vi "RTG_Host_Main.vi"() -> ()   [LabVIEW 2020]
uses:
  <vilib>/RTG/API/interface/public/State.ctl
  <vilib>/RTG/API/ip/common/host-types/Target Configuration.ctl
  <vilib>/RTG/API/ip/common/host-types/Synchronization - Host.ctl
  <vilib>/RTG/API/ip/common/host-types/Synchronization Mode - Host.ctl
  <vilib>/RTG/API/ip/common/host-types/Basic Target - Host.ctl
  <vilib>/RTG/API/ip/common/host-types/Target Motion Parameters.ctl
  <vilib>/RTG/API/ip/common/host-types/Single Target Motion Parameters.ctl
  <vilib>/RTG/API/interface/public/Coprocessor Link Status.ctl
  <vilib>/RTG/coprocessor/host/RTG Coprocessor Link Interface/Public/Coprocessor Status.ctl
  Controls/Enum/Program_Status_Enum.ctl
  Controls/Enum/RTG_Enum.ctl
  Controls/Enum/CoProcessor_Enum.ctl
  Controls/Enum/Supervisor_Enum.ctl
  Controls/Clust/RTG Clust.ctl
  <vilib>/RTG/API/interface/NI-RTG Interface.lvclass
  <vilib>/RTG/coprocessor/host/RTG Coprocessor Link Interface/RTG Coprocessor Link Interface.lvclass
  Controls/Clust/RTG API Clust.ctl
  support/Options - API Mode.ctl
  support/Options - Calibration.ctl
  support/Options - Remote.ctl
  <vilib>/Utility/error.llb/Error Cluster From Error Code.vi
  <vilib>/rvi/errors/niLvFpgaAdjustHostInterfaceError.vi
  <vilib>/rvi/interface/nirviReadWriteControl/nirviReadWriteControl.xnode
  RTG Examples.lvlib
  <vilib>/RTG/API/ip/common/host-types/Host Data Types v1.lvlib
  NiFpgaLv.dll
  <vilib>/rvi/interface/Simulation/niFpgaSimulationCallBeginRW.vi
panel:
  out "CoPr":i32
  out "RTG":i32
  out "Spvsr":i32
  out "Spvsr":T1=enum."Spvsr_InitCtrls"
  out "CoPr":T2
  out "RTG":T3
  out "App Status":T4
  in  "Tab Control":T5(tab)
  in  "Instrument Names":string[](array[string])=["5831_0"]
  in  "Coprocessor Names":string[](array[string])
  in  "Center Freqeuncies (Hz)":dbl[](array[numeric])=[5500000000.0] format="%#_6p"
  in  "Reference Levels (dBm)":dbl[](array[numeric])=[0.0]
  in  "Calibrate":bool=TRUE
  in  "abort system self cal":bool
  in  "Commit HW":bool
  in  "ExtAtten":dbl[](array[numeric]) caption="External Attenuations (dB)"
  in  "OffsFreq":dbl[](array[numeric]) caption="Offset Frequencies (Hz)" format="%#_6p"
  in  "ExtDelay":dbl[](array[numeric]) caption="External Delay (s)" format="%#_6p"
  in  "mmWave Radio Heads Enable":bool[](array[boolean])
  in  "PRI (s)":dbl[](array[numeric]) format="%#_6p"
  in  "Set PRIs":bool
  out "Min Latencies (s)":dbl[](array[numeric]) format="%#_6p"
  out "Min Common Attenuations (dB)":dbl[](array[numeric])
  out "Max Common Attenuations (dB)":dbl[](array[numeric])
  out "Versions":string[](array[string])
  in  "Common Attenuation (dB)":dbl
  in  "Auto Send Software Trigger":bool
  in  "Prepend Software Trigger":bool
  in  "Device Index":i32
  in  "Target Configuration Files":path[](array[path])
  in  "Target Configuration":T6 {"rtg targets"."time offset (s)" format="%#_6p"; "rtg targets"."doppler" format="%#_6p"}
  in  "Target Motion Parameters":T10={"target motions"=[{"target enable"=FALSE, "start time offset (s)"=-1e-09, "time offset rate of change (s/s)"=0.001, "start attenuation (dB)"=0.0, "attenuation rate of change (dB/s)"=0.0, "start frequency shift (Hz)"=0.0, "frequency shift rate of change (Hz/sec)"=0.0}], "scenario duration (s)"=67.0, "configuration update rate(Hz)"=15000.0} {"configuration update rate(Hz)" format="%#_6p"; "target motions"."frequency shift rate of change (Hz/sec)" format="%#_6p"; "target motions"."start frequency shift (Hz)" format="%#_6p"; "target motions"."time offset rate of change (s/s)" format="%#_6p"; "target motions"."start time offset (s)" format="%#_6p"}
  in  "Send TrgtCfg":bool
  in  "Send Motion":bool
  in  "Send Files":bool
  in  "Start RTG":bool
  in  "Stop RTG":bool
  in  "Send SW Trigg":bool
  out "rtg link status":T12[](array[typedef])
  out "Trigger Count":i32[][](array[numeric]) caption="Device Index vs Trigger Count"
  out "RTG Status":string
  out "RTG State":T13
  out "error out":errorcluster
  out "System Time":string
  out "coproc link":T14[](array[typedef]) caption="coprocessor link status"
  in  "Exit":bool
  # "v20230901"
  # "Configuration Files and Target Motion"
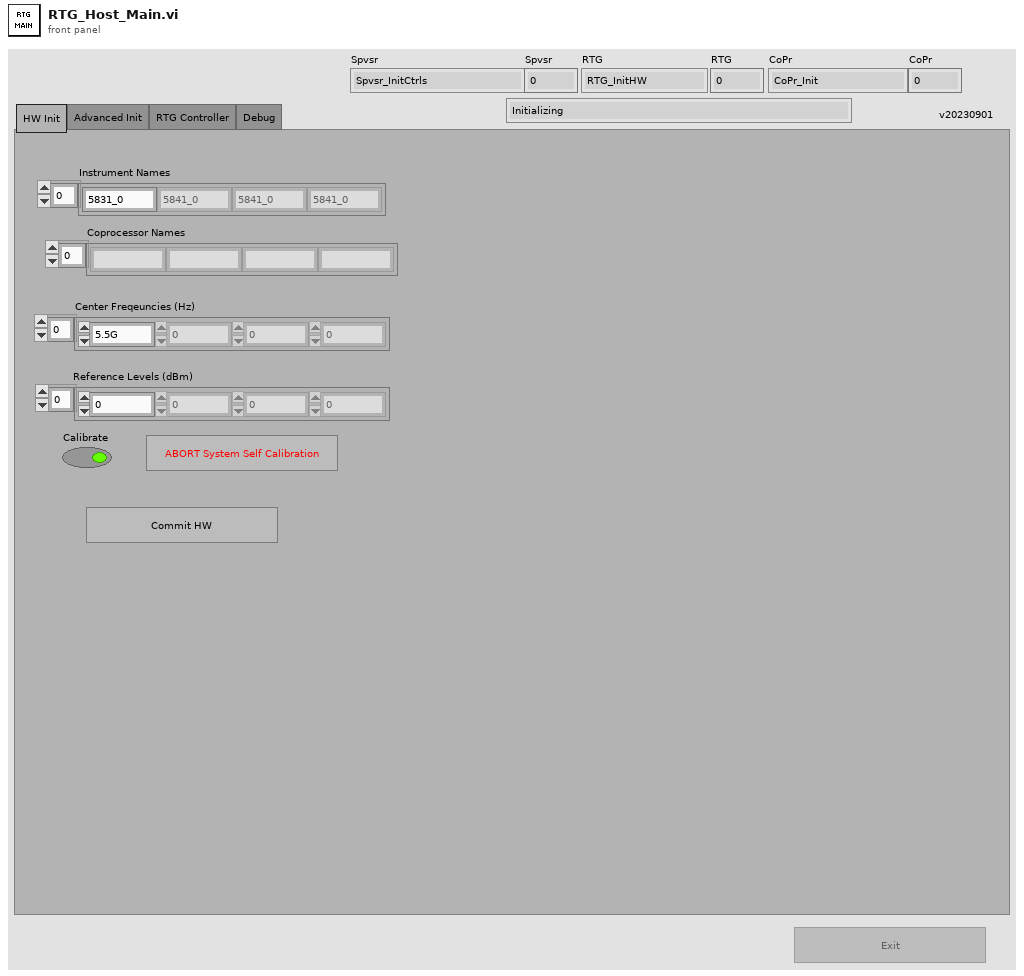
[diagram p1: front panel]
types:
  T1 = typedef "Supervisor_Enum.ctl" = enum16{"Spvsr_InitSW", "Spvsr_InitCtrls", "Spvsr_UpdtFP", "Spvsr_InitRTG", "Spvsr_StateCount", "Spvsr_Exit"}
  T2 = typedef "CoProcessor_Enum.ctl" = enum16{"CoPr_Init", "CoPr_Chk", "CoPr_Exit"}
  T3 = typedef "RTG_Enum.ctl" = enum16{"RTG_InitHW", "RTG_RefLvl", "RTG_mmWav", "RTG_Cal", "RTG_CalDone?", "RTG_ExtAtten", "RTG_GetCal", "RTG_SetPRIs", "RTG_CommAtten", "RTG_TargetSetup", "RTG_Send Files", "RTG_Send Target Cfg", "RTG_Send Motion", "RTG_Send SW Trigg", "RTG_Start", "RTG_Stop", "RTG_Chk", "RTG_Exit"}
  T4 = typedef "Program_Status_Enum.ctl" = enum16{"Initializing", "RTG Inactive", "Unconfigured", "RTG active", "Error", "Closing", "Closed"}
  T5 = enum32{"HW Init", "Advanced Init", "RTG Controller", "Debug"}
  T6 = typedef "Host Data Types v1.lvlib/Target Configuration.ctl" = cluster{"synchronization":T7, "rtg targets":T9[]}
  T7 = typedef "Host Data Types v1.lvlib/Synchronization - Host.ctl" = cluster{"synch mode":T8, "time offset (s)":dbl}
  T8 = typedef "Host Data Types v1.lvlib/Synchronization Mode - Host.ctl" = enum16{"Software Trigger", "Hardware Trigger", "Time Offset Relative to First", "Time Offset Relative to Last", "Pulse Rising Edge", "Pulse Falling Edge"}
  T9 = typedef "Host Data Types v1.lvlib/Basic Target - Host.ctl" = cluster{"time offset (s)":dbl, "attenuaton (dB)":dbl, "doppler":dbl, "target enable":bool, "relative velocity enable":bool}
  T10 = typedef "Host Data Types v1.lvlib/Target Motion Parameters.ctl" = cluster{"target motions":T11[], "scenario duration (s)":dbl, "configuration update rate(Hz)":dbl}
  T11 = typedef "Host Data Types v1.lvlib/Single Target Motion Parameters.ctl" = cluster{"target enable":bool, "start time offset (s)":dbl, "time offset rate of change (s/s)":dbl, "start attenuation (dB)":dbl, "attenuation rate of change (dB/s)":dbl, "start frequency shift (Hz)":dbl, "frequency shift rate of change (Hz/sec)":dbl}
  T12 = typedef "NI-RTG v1.lvlib/NI-RTG Interface.lvclass/Coprocessor Link Status.ctl" = cluster{"task name":string, "device name":string, "hard error":bool, "soft error":bool, "channel up":bool, "system reset":bool}
  T13 = typedef "NI-RTG v1.lvlib/NI-RTG Interface.lvclass/State.ctl" = enum16{"Idle", "Inactive", "Active", "System Self Calibration"}
  T14 = typedef "RTG Coprocessor Link Interface v1 Host.lvlib/RTG Coprocessor Link Interface.lvclass/Coprocessor Status.ctl" = cluster{"tx read count":u64, "tx read overflow":bool, "rx read count":u64, "rx read overflow":bool}
  T15 = cluster{"CoPr Refs":refnum<class "RTG Coprocessor Link Interface.lvclass">[]}
  T16 = typedef "RTG Clust.ctl" = cluster{"VST_Names":string[], "OptionString":string, "RTG Ref":refnum<class "NI-RTG Interface.lvclass">, "Index":i32, "AutoSend":bool, "Prepend":bool, "state":T13}
  T17 = enum8{"Enabled", "Disabled", "Disabled and Grayed Out"}
  T18 = typedef "RTG API Clust.ctl" = cluster{"Local?":T19, "Cal":T20, "Remote":T21, "ini path":path}
  T19 = typedef "RTG Examples.lvlib/Options - API Mode.ctl" = enum16{"Local", "Remote"}
  T20 = typedef "RTG Examples.lvlib/Options - Calibration.ctl" = cluster{"enable internal loopback  ":bool, "enable overwrite cal data  ":bool, "enable save cal data           ":bool, "disable self cal range          ":bool}
  T21 = typedef "RTG Examples.lvlib/Options - Remote.ctl" = cluster{"ip address":string, "port":string, "certificate path":path, "timeout (ms)":i32}
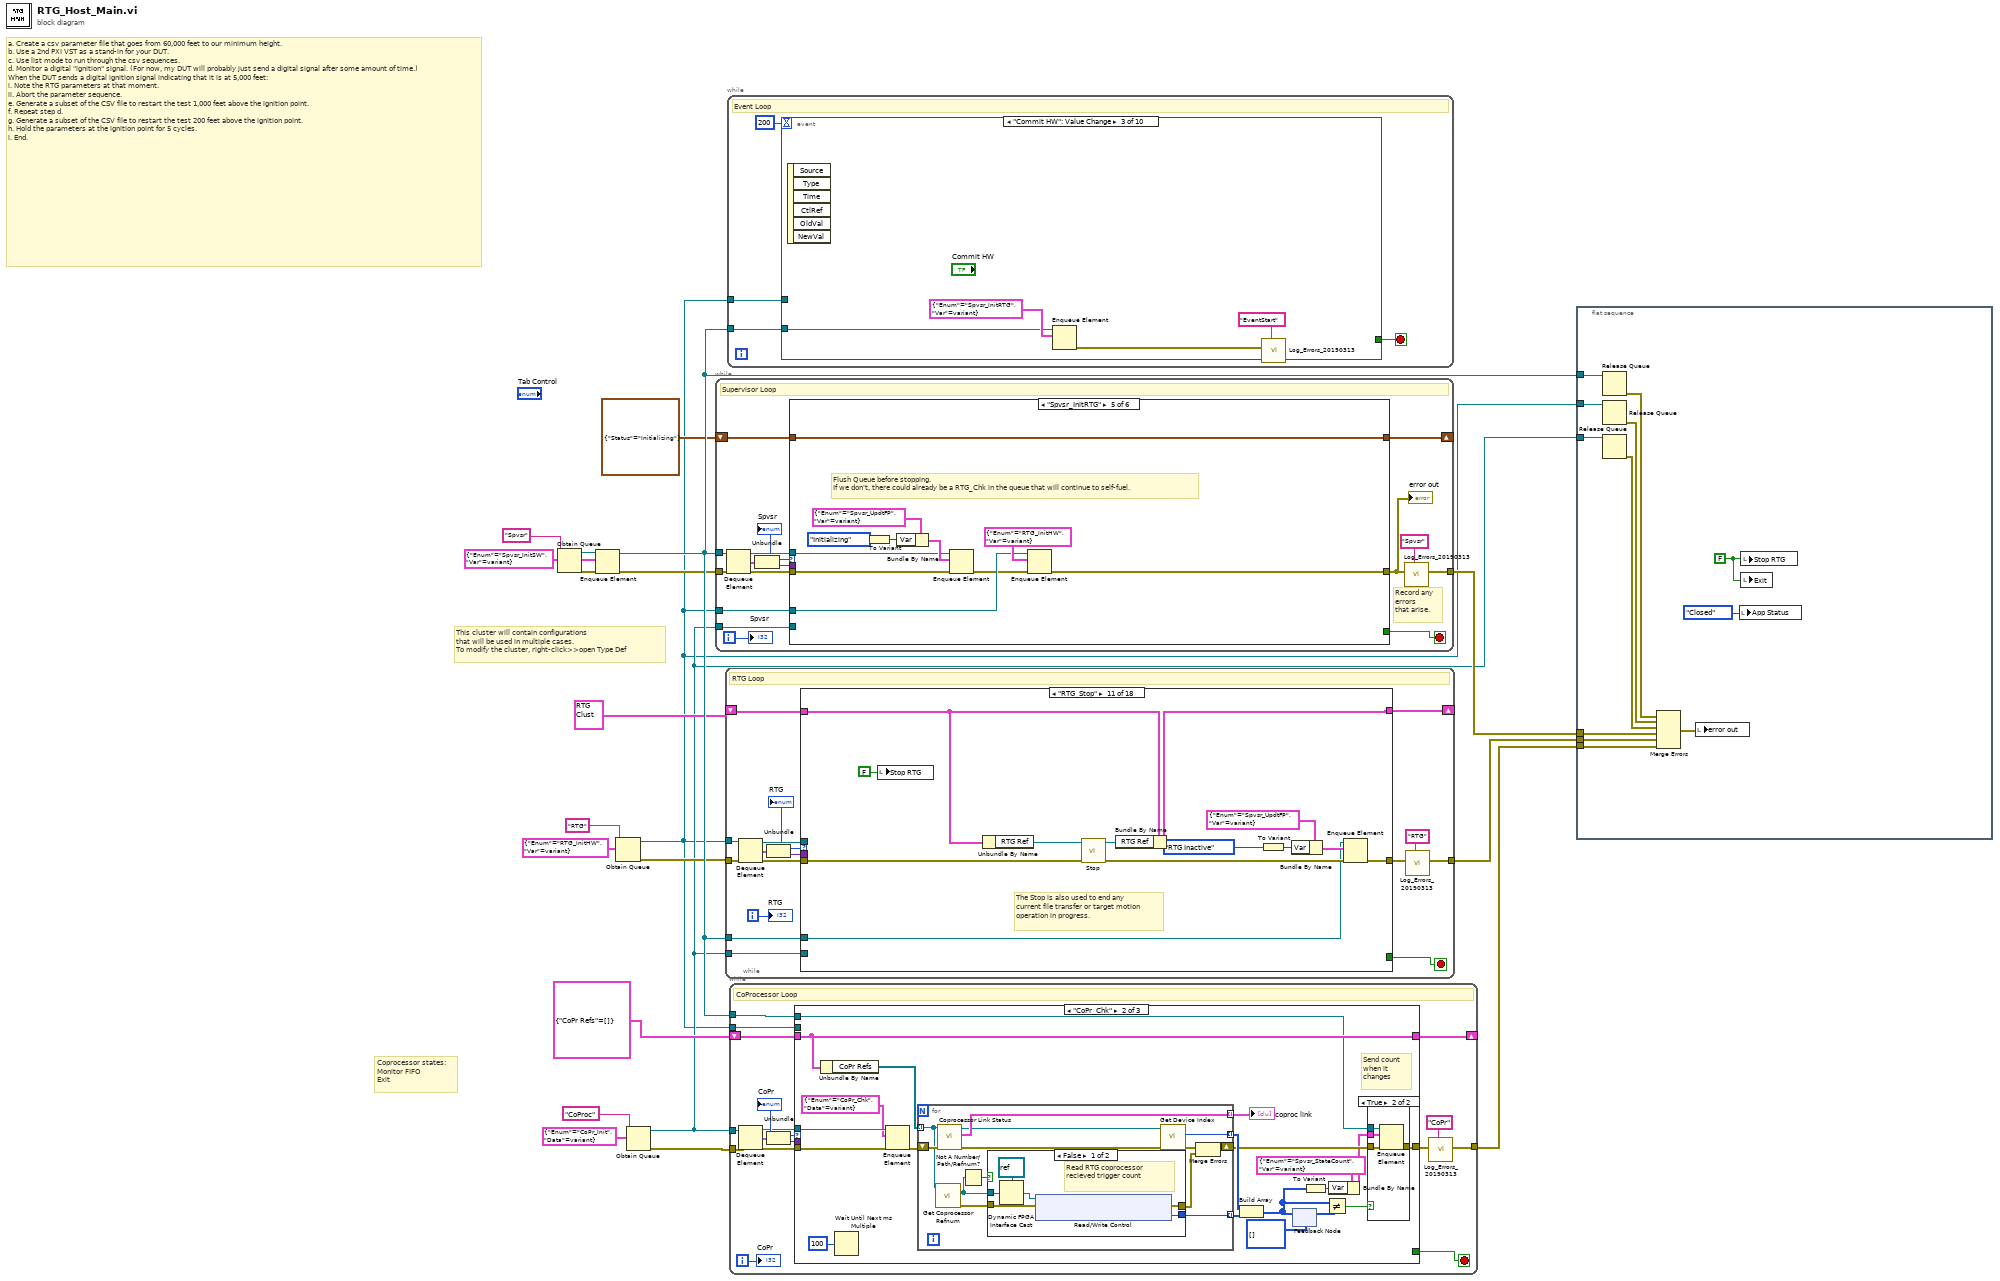
[diagram p0: block diagram]
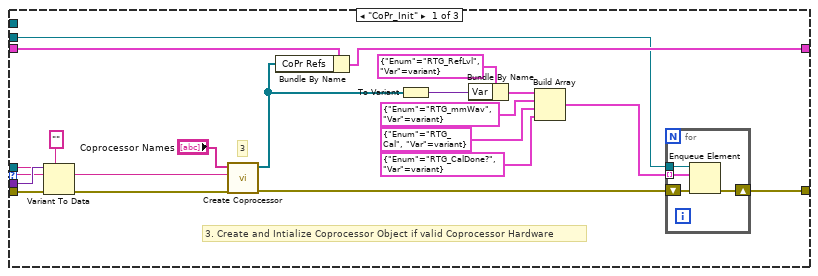
[diagram p2: hidden frame]
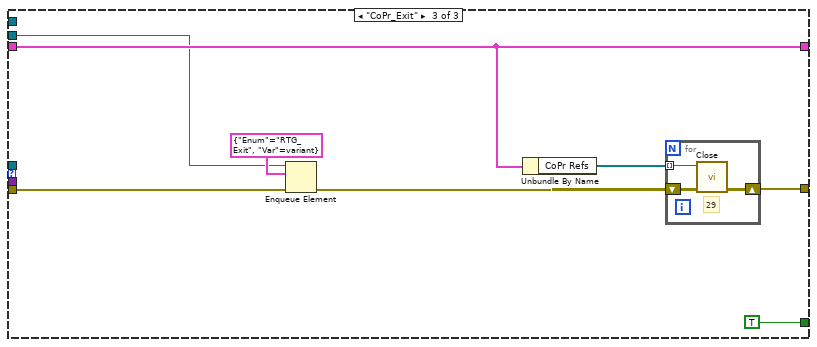
[diagram p5: hidden frame]
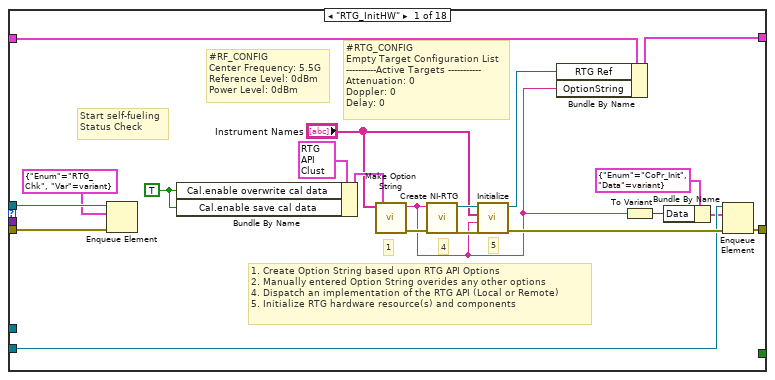
[diagram p6: hidden frame]
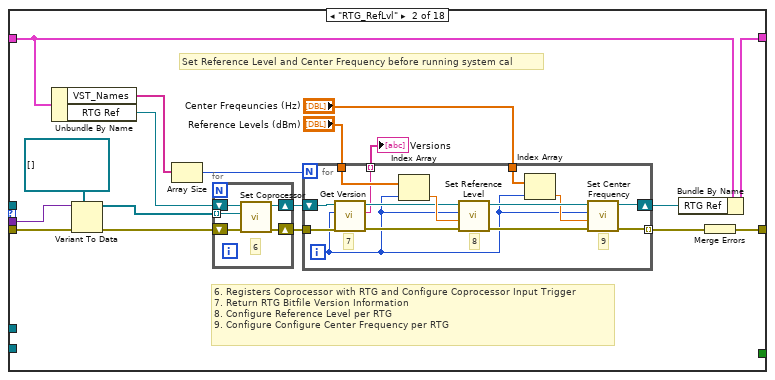
[diagram p7: hidden frame]
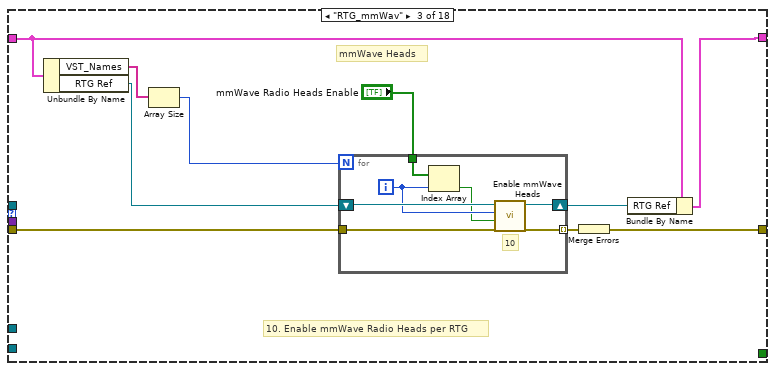
[diagram p8: hidden frame]
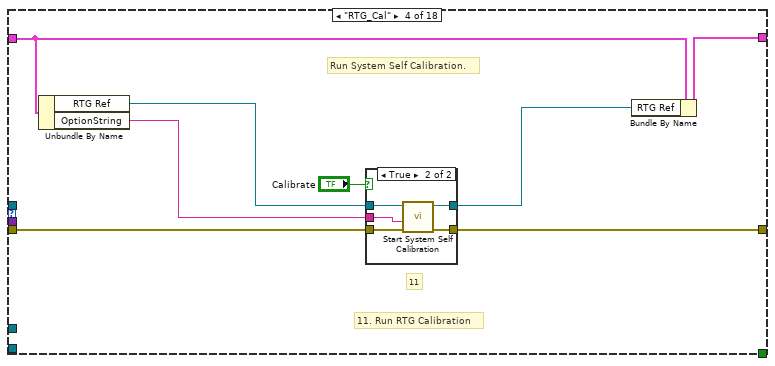
[diagram p9: hidden frame]
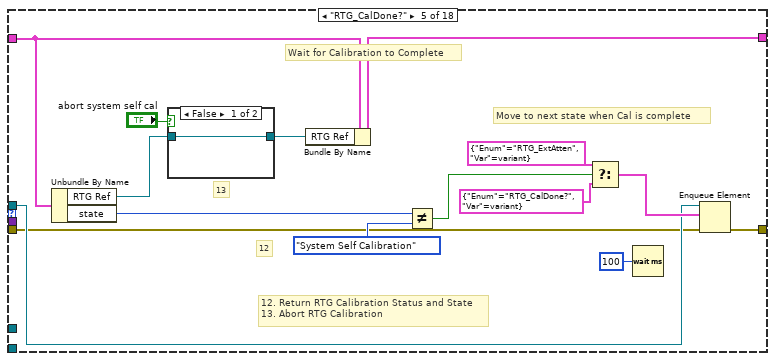
[diagram p11: hidden frame]
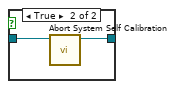
[diagram p12: hidden frame]
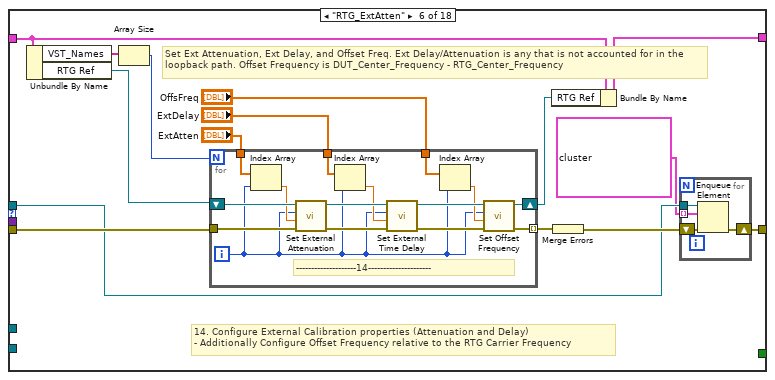
[diagram p13: hidden frame]
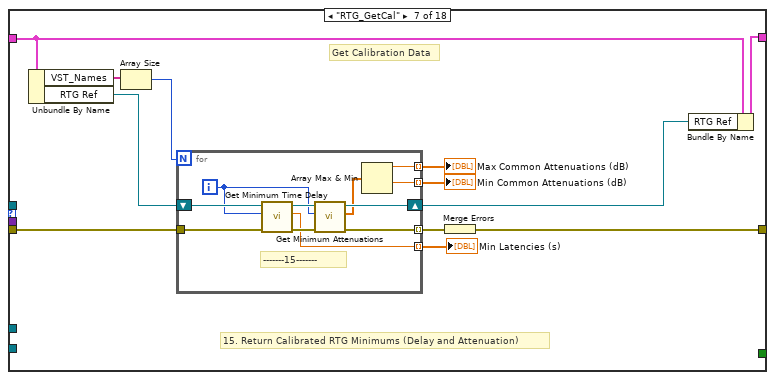
[diagram p14: hidden frame]
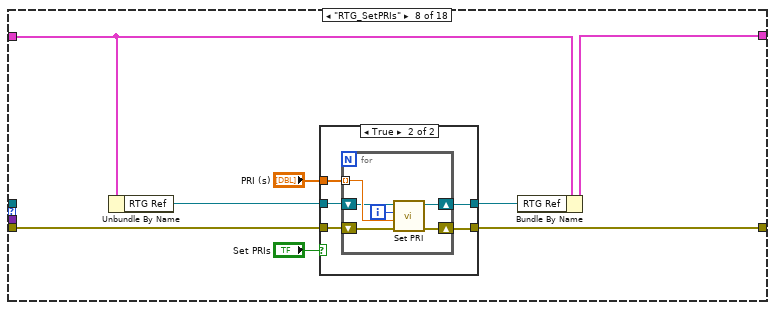
[diagram p15: hidden frame]
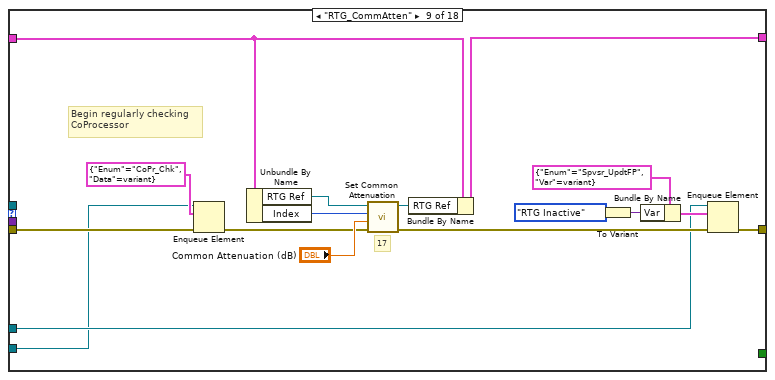
[diagram p17: hidden frame]
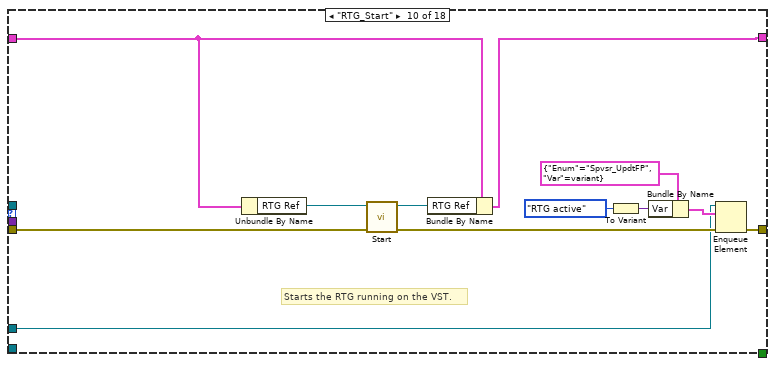
[diagram p18: hidden frame]
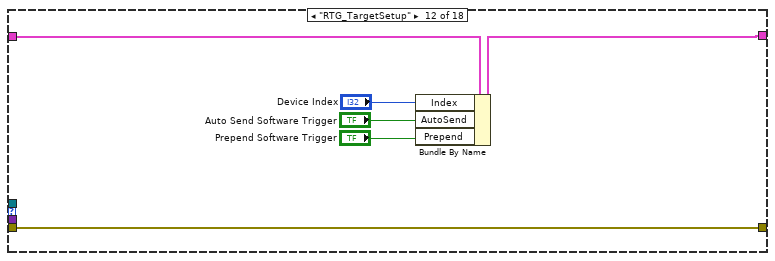
[diagram p19: hidden frame]
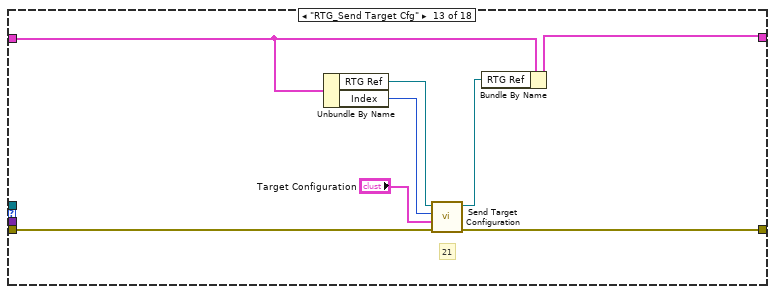
[diagram p20: hidden frame]
diagram:
  w16 = cluster{"Enum":T1, "Var":variant} {"Enum"=enum."Spvsr_InitSW", "Var"=variant}
  # "Coprocessor states:\nMonitor FIFO\nExit"
  # "a.\tCreate a csv parameter file that goes from 60,000 feet to our minimum height. \nb.\tUse a 2nd PXI VST as a stand-in for your DUT.\nc.\tUse list mode to run through the csv sequences.\nd.\tMonitor a digital \"ignition\" signal. (For now, my DUT will probably just send a digital signal after some amount of time.) When the DUT sends a digital ignition signal indicating that it is at 5,000 feet:\ni.\tNote the RTG parameters at that moment.\nii.\tAbort the parameter sequence.\ne.\tGenerate a subset of the CSV file to restart the test 1,000 feet above the ignition point.\nf.\tRepeat step d.\ng.\tGenerate a subset of the CSV file to restart the test 200 feet above the ignition point.\nh.\tHold the parameters at the ignition point for 5 cycles.\ni.\tEnd."
  # "This cluster will contain configurations\nthat will be used in multiple cases.\nTo modify the cluster, right-click>>open Type Def"
  n1 = Obtain Queue(name (unnamed)="Spvsr", element data type=w16) -> (queue out=w17:refnum<queue>, error out=w19:errorcluster)  [unwired: 3 in, 1 out]
  n2 = Enqueue Element(queue=w17, element=w16, error in (no error)=w19) -> (queue out=w20:refnum<queue>, error out=w18:errorcluster)  [unwired: 1 in, 1 out]
  n3 = Obtain Queue(name (unnamed)="RTG", element data type=cluster{"Enum":T3, "Var":variant} {"Enum"=enum."RTG_InitHW", "Var"=variant}) -> (queue out=w1:refnum<queue>, error out=w14:errorcluster)  [unwired: 3 in, 1 out]
  n4 = Obtain Queue(name (unnamed)="CoProc", element data type=cluster{"Enum":T2, "Data":variant} {"Enum"=enum."CoPr_Init", "Data"=variant}) -> (queue out=w2:refnum<queue>, error out=w12:errorcluster)  [unwired: 3 in, 1 out]
  n5 = while {
    tunnel: w18 -> [w36]
    tunnel: w20 -> [w34]
    tunnel: w1 -> [w29]
    tunnel: [w26] -> w6
    tunnel: w2 -> [w25]
    shift-right: [w23] -> _
    shift-left: cluster{"Status":T4} {"Status"=enum."Initializing"} -> [w24]
    i -> [w21]
    stop <- w22 stop-if-true
    # "Record any\nerrors \nthat arise."
    # "Supervisor Loop"
    n6 = Dequeue Element(queue=w34, error in (no error)=w36) -> (queue out=w32:refnum<queue>, element=w33:cluster{"Enum":T1, "Var":variant}, error out=w35:errorcluster)  [unwired: 1 in, 1 out]
    n7 = Unbundle(w33) -> ("Enum"=w31:T1, "Var"=w30:variant)
    "Spvsr" <- w31
    n8 = case shown="\"Spvsr_InitRTG\"" w31 {
      tunnel: w35 -> [w49 w51 w62 w124 w130 w142]
      tunnel: w32 -> [w48 w50 _ _ w127 _]
      tunnel: w30 -> [_ _ w61 _ _ w140]
      tunnel: w29 -> [_ _ _ w122 w136 _]
      tunnel: [w43 w52 w64 w121 w128 w138] -> w27
      tunnel: w25 -> [_ _ _ w119 _ _]
      tunnel: w24 -> [w46 w57 w77 w115 w135 w143]
      tunnel: [w45 w57 w77 w115 w135 w143] -> w23
      tunnel: [_ _ _ TRUE _ _] -> w22
      frame "Spvsr_InitSW" {
        n9 = Enqueue Element(queue=w48, element=cluster{"Enum":T1, "Var":variant} {"Enum"=enum."Spvsr_InitCtrls", "Var"=variant}, error in (no error)=w49) -> (queue out=w41:refnum<queue>, error out=w42:errorcluster)  [unwired: 1 in, 1 out]
        n10 = Bundle By Name(cluster=w46, "Status"=Program_Status_Enum."Initializing") -> (w45:cluster{"Status":T4})
        n11 = To Variant(anything=Program_Status_Enum."Initializing" ("Status")) -> (Variant=w38:variant)
        n12 = Bundle By Name(cluster=cluster{"Enum":T1, "Var":variant} {"Enum"=enum."Spvsr_UpdtFP", "Var"=variant}, "Var"=w38) -> (w37:cluster{"Enum":T1, "Var":variant})
        n13 = Enqueue Element(queue=w41, element=w37, error in (no error)=w42) -> (error out=w43:errorcluster)  [unwired: 1 in, 2 out]
      }
      frame "Spvsr_InitCtrls" {
        w58 = FALSE ("Exit")
        n14 = To Variant(anything=Program_Status_Enum."Unconfigured" ("Status")) -> (Variant=w56:variant)
        n15 = Bundle By Name(cluster=cluster{"Enum":T1, "Var":variant} {"Enum"=enum."Spvsr_UpdtFP", "Var"=variant}, "Var"=w56) -> (w54:cluster{"Enum":T1, "Var":variant})
        n16 = Enqueue Element(queue=w50, element=w54, error in (no error)=w51) -> (error out=w52:errorcluster)  [unwired: 1 in, 2 out]
        n17 = local write "Exit"(w58) -> ()
        n18 = local write "Stop RTG"(w58) -> ()
      }
      frame "Spvsr_UpdtFP" {
        n19 = Variant To Data(error in=w62, type=Program_Status_Enum."Closed" ("App Status"), Variant=w61) -> (data=w59:T4, error out=w63:errorcluster)
        "App Status" <- w59
        n20 = case shown="\"Unconfigured\"" w59 {
          tunnel: [T17."Disabled and Grayed Out" ("Disabled") T17."Enabled" ("Disabled") T17."Disabled and Grayed Out" ("Disabled") T17."Disabled and Grayed Out" ("Disabled") T17."Enabled" ("Disabled") T17."Disabled and Grayed Out" ("Disabled")] -> w70
          tunnel: [T17."Disabled and Grayed Out" ("Disabled") T17."Enabled" ("Disabled") T17."Disabled and Grayed Out" ("Disabled") T17."Disabled and Grayed Out" ("Disabled") T17."Disabled and Grayed Out" ("Disabled") T17."Enabled" ("Disabled")] -> w69
          tunnel: [T17."Enabled" ("Disabled") T17."Enabled" ("Disabled") T17."Disabled and Grayed Out" ("Disabled") T17."Enabled" ("Disabled") T17."Enabled" ("Disabled") T17."Enabled" ("Disabled")] -> w68
          tunnel: [T17."Disabled and Grayed Out" ("Disabled") T17."Disabled and Grayed Out" ("Disabled") T17."Disabled and Grayed Out" ("Disabled") T17."Disabled and Grayed Out" ("Disabled") T17."Disabled and Grayed Out" ("Disabled") T17."Enabled" ("Disabled")] -> w67
          tunnel: [T17."Disabled and Grayed Out" ("Disabled") T17."Disabled and Grayed Out" ("Disabled") T17."Disabled and Grayed Out" ("Disabled") T17."Disabled and Grayed Out" ("Disabled") T17."Disabled and Grayed Out" ("Disabled") T17."Enabled" ("Disabled")] -> w66
          tunnel: [T17."Disabled and Grayed Out" ("Disabled") T17."Disabled and Grayed Out" ("Disabled") T17."Disabled and Grayed Out" ("Disabled") T17."Disabled and Grayed Out" ("Disabled") T17."Disabled and Grayed Out" ("Disabled") T17."Enabled" ("Disabled")] -> w65
          frame "Unconfigured" {
          }
          frame "Error" {
          }
          frame "Closing", "Closed" {
          }
          frame "Initializing" {
          }
          frame "RTG Inactive" {
          }
          frame "RTG active" {
          }
        }
        n21 = property on="Start RTG" class="Bool"(error in=w63, "DisabledEnum"=w70) -> (error out=w71:errorcluster)  [unwired: 1 in, 1 out]
        n22 = property on="Stop RTG" class="Bool (strict)"("DisabledEnum"=w69) -> (error out=w72:errorcluster)  [unwired: 2 in, 1 out]
        n23 = property on="Exit" class="Bool (strict)"("DisabledEnum"=w68) -> (error out=w73:errorcluster)  [unwired: 2 in, 1 out]
        n24 = property on="Send TrgtCfg" class="Bool"("DisabledEnum"=w67) -> (error out=w74:errorcluster)  [unwired: 2 in, 1 out]
        n25 = property on="Send Motion" class="Bool"("DisabledEnum"=w66) -> (error out=w75:errorcluster)  [unwired: 2 in, 1 out]
        n26 = property on="Send Files" class="Bool"("DisabledEnum"=w65) -> (error out=w76:errorcluster)  [unwired: 2 in, 1 out]
        n27 = Merge Errors(w71, w72, w73, w74, w75, w76) -> (w64:errorcluster)
      }
      frame "Spvsr_Exit" {
        # "RTG Exit is called from Coprocesor Exit\nto prevent a race condition"
        # "Flush Queue before stopping.\nIf we don't, there could already be a RTG_Chk in the queue that will continue to self-fuel."
        n28 = Flush Queue(queue=w122, error in (no error)=w124) -> (queue out=w123:refnum<queue>, error out=w125:errorcluster)  [unwired: 1 out]
        n29 = Enqueue Element(queue=w123, element=cluster{"Enum":T3, "Var":variant} {"Enum"=enum."RTG_Stop", "Var"=variant}, error in (no error)=w125) -> (error out=w117:errorcluster)  [unwired: 1 in, 2 out]
        n30 = Flush Queue(queue=w119, error in (no error)=w117) -> (queue out=w118:refnum<queue>, error out=w116:errorcluster)  [unwired: 1 out]
        n31 = Enqueue Element(queue=w118, element=cluster{"Enum":T2, "Data":variant} {"Enum"=enum."CoPr_Exit", "Data"=variant}, error in (no error)=w116) -> (error out=w121:errorcluster)  [unwired: 1 in, 2 out]
      }
      frame "Spvsr_InitRTG" {
        # "Flush Queue before stopping.\nIf we don't, there could already be a RTG_Chk in the queue that will continue to self-fuel."
        n32 = To Variant(anything=Program_Status_Enum."Initializing" ("Status")) -> (Variant=w134:variant)
        n33 = Bundle By Name(cluster=cluster{"Enum":T1, "Var":variant} {"Enum"=enum."Spvsr_UpdtFP", "Var"=variant}, "Var"=w134) -> (w132:cluster{"Enum":T1, "Var":variant})
        n34 = Enqueue Element(queue=w127, element=w132, error in (no error)=w130) -> (error out=w129:errorcluster)  [unwired: 1 in, 2 out]
        n35 = Enqueue Element(queue=w136, element=cluster{"Enum":T3, "Var":variant} {"Enum"=enum."RTG_InitHW", "Var"=variant}, error in (no error)=w129) -> (error out=w128:errorcluster)  [unwired: 1 in, 2 out]
      }
      frame "Spvsr_StateCount" {
        # "Making this value available to the rest of the program."
        n36 = Variant To Data(error in=w142, type=i32[][] [] ("appended array"), Variant=w140) -> (data=→"Trigger Count":i32[][], error out=w138:errorcluster)
      }
    }
    "error out" <- w27
    n37 = call "Log_Errors_20190313.vi"("LoopName"="Spvsr", "error in"=w27) -> ("error out"=w26:errorcluster)  [unwired: 9 in]
    "Spvsr" <- w21
  }
  n38 = while {
    tunnel: w14 -> [w159]
    shift-right: [w151] -> _
    shift-left: T16 {"VST_Names"=["5841_0"], "OptionString"="", "RTG Ref"=refnum, "Index"=0, "AutoSend"=FALSE, "Prepend"=FALSE, "state"=enum."Idle"} ("DAQ Clust") -> [w152]
    tunnel: [w149] -> w5
    tunnel: w2 -> [w148]
    tunnel: w1 -> [w145]
    tunnel: w20 -> [w144]
    i -> [w146]
    stop <- w147 stop-if-true
    # "RTG Loop"
    n39 = Dequeue Element(queue=w145, error in (no error)=w159) -> (queue out=w156:refnum<queue>, element=w157:cluster{"Enum":T3, "Var":variant}, error out=w158:errorcluster)  [unwired: 1 in, 1 out]
    n40 = Unbundle(w157) -> ("Enum"=w155:T3, "Var"=w154:variant)
    "RTG" <- w155
    n41 = case shown="\"RTG_Stop\"" w155 {
      tunnel: w158 -> [w162 w188 w221 w238 w250 w276 w305 w327 w346 w373 w382 w392 w399 w407 w436 w463 w475 w485]
      tunnel: w156 -> [w161 _ _ _ w253 w268 _ _ _ _ _ _ _ _ _ _ w474 _]
      tunnel: w154 -> [_ w185 _ _ _ _ _ _ _ _ _ _ _ _ _ _ _ _]
      tunnel: w152 -> [w179 w182 w217 w241 w263 w281 w311 w331 w361 w369 w385 w390 w396 w414 w443 w465 w480 w482]
      tunnel: [w178 w181 w218 w240 w262 w280 w312 w330 w360 w370 w386 w391 w395 w413 w442 w464 w479 w482] -> w151
      tunnel: [w168 w183 w220 w237 w252 w269 w304 w326 w352 w363 w375 w392 w398 w406 w435 w462 w469 w484] -> w150
      tunnel: w148 -> [w167 _ _ _ _ _ _ _ w345 _ _ _ _ _ _ _ _ _]
      tunnel: [_ _ _ _ _ _ _ _ _ _ _ _ _ _ _ _ _ TRUE] -> w147
      tunnel: w144 -> [_ _ _ _ _ _ _ _ w349 w362 w374 _ _ _ _ _ _ _]
      frame "RTG_InitHW" {
        w177 = TRUE ("Calibration Options.enable overwrite cal data")
        # "Start self-fueling\nStatus Check"
        # "1. Create Option String based upon RTG API Options\n2. Manually entered Option String overides any other options\n4. Dispatch an implementation of the RTG API (Local or Remote)\n5. Initialize RTG hardware resource(s) and components"
        # "#RTG_CONFIG\nEmpty Target Configuration List\n----------Active Targets -----------\nAttenuation: 0\nDoppler: 0\nDelay: 0"
        # "#RF_CONFIG\nCenter Frequency: 5.5G\nReference Level: 0dBm\nPower Level: 0dBm"
        # "4"
        # "1"
        # "5"
        n42 = Enqueue Element(queue=w161, element=cluster{"Enum":T3, "Var":variant} {"Enum"=enum."RTG_Chk", "Var"=variant}, error in (no error)=w162) -> ()  [unwired: 1 in, 3 out]
        n43 = Bundle By Name(cluster=T18 {"Local?"=enum."Local", "Cal"={"enable internal loopback  "=FALSE, "enable overwrite cal data  "=FALSE, "enable save cal data           "=FALSE, "disable self cal range          "=FALSE}, "Remote"={"ip address"="", "port"="50052", "certificate path"=path "", "timeout (ms)"=15000}, "ini path"=path ""} ("RTG API Options"), "Cal.enable overwrite cal data"=w177, "Cal.enable save cal data"=w177) -> (w176:T18)
        n44 = call "Make Option String.vi"("RTG API Options"=w176, "instrument names"="Instrument Names") -> ("error out"=w175:errorcluster, "option string"=w165:string)  [unwired: 8 in]
        n45 = call <vilib>:"Create NI-RTG.vi"("error in"=w175, "option string"=w165) -> ("error out"=w173:errorcluster, "NI-RTG Interface out"=w172:refnum<class "NI-RTG Interface.lvclass">)  [unwired: 8 in]
        n46 = call-dynamic "Initialize.vi"("error in"=w173, "option string"=w165, "instrument names"="Instrument Names", "ni-rtg interface"=w172) -> ("error out"=w169:errorcluster, "ni-rtg interface out"=w170:refnum<class "NI-RTG Interface.lvclass">)  [unwired: 6 in]
        n47 = Bundle By Name(cluster=w179, "RTG Ref"=w170, "OptionString"=w165) -> (w178:T16)
        n48 = To Variant(anything=w165) -> (Variant=w164:variant)
        n49 = Bundle By Name(cluster=cluster{"Enum":T2, "Data":variant} {"Enum"=enum."CoPr_Init", "Data"=variant}, "Data"=w164) -> (w163:cluster{"Enum":T2, "Data":variant})
        n50 = Enqueue Element(queue=w167, element=w163, error in (no error)=w169) -> (error out=w168:errorcluster)  [unwired: 1 in, 2 out]
      }
      frame "RTG_RefLvl" {
        # "6. Registers Coprocessor with RTG and Configure Coprocessor Input Trigger\n7. Return RTG Bitfile Version Information\n8. Configure Reference Level per RTG\n9. Configure Configure Center Frequency per RTG"
        # "Set Reference Level and Center Frequency before running system cal"
        n51 = Unbundle By Name(w182) -> ("VST_Names"=w190:string[], "RTG Ref"=w191:refnum<class "NI-RTG Interface.lvclass">)
        n52 = Variant To Data(error in=w188, type=refnum<class "RTG Coprocessor Link Interface.lvclass">[] [] ("rtg coprocessor links"), Variant=w185) -> (data=w184:refnum<class "RTG Coprocessor Link Interface.lvclass">[], error out=w187:errorcluster)
        n53 = Array Size(array=w190) -> (size(s)=w189:i32)
        n54 = for {
          shift-right: [w216] -> w195
          shift-left: w187 -> [w214]
          shift-right: [w215] -> w196
          shift-left: w191 -> [w213]
          tunnel: w184 -> [w212] mode=indexing
          # "6"
          n55 = call-dynamic "Set Coprocessor.vi"("error in"=w214, "rtg coprocessor link interface"=w212, "rtg api interface"=w213) -> ("error out"=w216:errorcluster, "rtg api interface out"=w215:refnum<class "NI-RTG Interface.lvclass">)  [unwired: 7 in]
        }
        n56 = for {
          N: w189 -> [_]
          tunnel: w195 -> [w201]
          tunnel: "Reference Levels (dBm)" -> [w209]
          tunnel: "Center Freqeuncies (Hz)" -> [w207]
          shift-right: [w205] -> w180
          shift-left: w196 -> [w203]
          tunnel: [w204] -> w194 mode=indexing
          tunnel: [w198] -> w197 mode=indexing
          i -> [w199]
          # "9"
          # "8"
          # "7"
          n57 = call-dynamic "Get Version.vi"("error in"=w201, "device index (0)"=w199, "NI-RTG Interface in"=w203) -> ("error out"=w200:errorcluster, "version"=w198:string, "NI-RTG Interface out"=w202:refnum<class "NI-RTG Interface.lvclass">)  [unwired: 6 in]
          n58 = Index Array(array=w209, index=w199) -> (element=w208:dbl)
          n59 = call-dynamic "Set Reference Level.vi"("error in"=w200, "reference level (dBm)"=w208, "device index (0)"=w199, "rtg api interface"=w202) -> ("error out"=w210:errorcluster, "rtg api interface out"=w211:refnum<class "NI-RTG Interface.lvclass">)  [unwired: 6 in]
          n60 = Index Array(array=w207, index=w199) -> (element=w206:dbl)
          n61 = call-dynamic "Set Center Frequency.vi"("error in"=w210, "center frequency (Hz)"=w206, "device index (0)"=w199, "rtg api interface"=w211) -> ("error out"=w204:errorcluster, "rtg api interface out"=w205:refnum<class "NI-RTG Interface.lvclass">)  [unwired: 6 in]
        }
        "Versions" <- w197
        n62 = Bundle By Name(cluster=w182, "RTG Ref"=w180) -> (w181:T16)
        n63 = Merge Errors(w194) -> (w183:errorcluster)
      }
      frame "RTG_mmWav" {
        # "10. Enable mmWave Radio Heads per RTG"
        # "mmWave Heads"
        n64 = Unbundle By Name(w217) -> ("VST_Names"=w226:string[], "RTG Ref"=w223:refnum<class "NI-RTG Interface.lvclass">)
        n65 = Array Size(array=w226) -> (size(s)=w222:i32)
        n66 = for {
          N: w222 -> [_]
          shift-right: [w230] -> w219
          shift-left: w223 -> [w231]
          tunnel: w221 -> [w233]
          tunnel: [w232] -> w224 mode=indexing
          tunnel: "mmWave Radio Heads Enable" -> [w229]
          i -> [w228]
          # "10"
          n67 = Index Array(array=w229, index=w228) -> (element=w227:bool)
          n68 = call-dynamic "Enable mmWave Heads.vi"("error in"=w233, "enable mmWave"=w227, "device index (0)"=w228, "ni-rtg interface"=w231) -> ("error out"=w232:errorcluster, "ni-rtg interface out"=w230:refnum<class "NI-RTG Interface.lvclass">)  [unwired: 6 in]
        }
        n69 = Merge Errors(w224) -> (w220:errorcluster)
        n70 = Bundle By Name(cluster=w217, "RTG Ref"=w219) -> (w218:T16)
      }
      frame "RTG_Cal" {
        # "11"
        # "11. Run RTG Calibration"
        # "Run System Self Calibration."
        n71 = Unbundle By Name(w241) -> ("RTG Ref"=w236:refnum<class "NI-RTG Interface.lvclass">, "OptionString"=w234:string)
        n72 = case shown="True" "Calibrate" {
          tunnel: w236 -> [w243 w248]
          tunnel: w238 -> [w242 w247]
          tunnel: [w243 w246] -> w235
          tunnel: [w242 w245] -> w237
          tunnel: w234 -> [_ w244]
          frame False {
          }
          frame True {
            n73 = call-dynamic "Start System Self Calibration.vi"("error in"=w247, "option string"=w244, "rtg api interface"=w248) -> ("error out"=w245:errorcluster, "rtg api interface out"=w246:refnum<class "NI-RTG Interface.lvclass">)  [unwired: 7 in]
          }
        }
        n74 = Bundle By Name(cluster=w241, "RTG Ref"=w235) -> (w240:T16)
      }
      frame "RTG_CalDone?" {
        # "Move to next state when Cal is complete"
        # "13"
        # "12"
        # "12. Return RTG Calibration Status and State\n13. Abort RTG Calibration"
        # "Wait for Calibration to Complete"
        n75 = Unbundle By Name(w263) -> ("RTG Ref"=w261:refnum<class "NI-RTG Interface.lvclass">, "state"=w249:T13)
        n76 = case shown="False" "abort system self cal" {
          tunnel: w261 -> [w264 w266]
          tunnel: [w264 w265] -> w251
          frame False {
          }
          frame True {
            n77 = call-dynamic "Abort System Self Calibration.vi"("rtg-api interface"=w266) -> ("rtg-api interface out"=w265:refnum<class "NI-RTG Interface.lvclass">)  [unwired: 9 in, 1 out]
          }
        }
        n78 = Bundle By Name(cluster=w263, "RTG Ref"=w251) -> (w262:T16)
        n79 = Not Equal?(x=w249, y=State."System Self Calibration") -> (x != y?=w254:bool)
        n80 = Select(t=cluster{"Enum":T3, "Var":variant} {"Enum"=enum."RTG_ExtAtten", "Var"=variant} ("element"), s=w254, f=cluster{"Enum":T3, "Var":variant} {"Enum"=enum."RTG_CalDone?", "Var"=variant} ("element")) -> (s? t:f=w257:cluster{"Enum":T3, "Var":variant})
        n81 = Wait (ms)(milliseconds to wait=u32 100) -> ()  [unwired: 1 out]
        n82 = Enqueue Element(queue=w253, element=w257, error in (no error)=w250) -> (error out=w252:errorcluster)  [unwired: 1 in, 2 out]
      }
      frame "RTG_ExtAtten" {
        # "Set Ext Attenuation, Ext Delay, and Offset Freq. Ext Delay/Attenuation is any that is not accounted for in the loopback path. Offset Frequency is DUT_Center_Frequency - RTG_Center_Frequency"
        # "14. Configure External Calibration properties (Attenuation and Delay)\n- Additionally Configure Offset Frequency relative to the RTG Carrier Frequency"
        n83 = Unbundle By Name(w281) -> ("VST_Names"=w279:string[], "RTG Ref"=w272:refnum<class "NI-RTG Interface.lvclass">)
        n84 = Array Size(array=w279) -> (size(s)=w273:i32)
        n85 = for {
          N: w273 -> [_]
          shift-right: [w290] -> w271
          shift-left: w272 -> [w300]
          tunnel: "ExtAtten" -> [w298]
          tunnel: "ExtDelay" -> [w296]
          tunnel: [w292] -> w275 mode=indexing
          tunnel: w276 -> [w289]
          tunnel: "OffsFreq" -> [w288]
          i -> [w286]
          # "--------------------14---------------------"
          n86 = Index Array(array=w298, index=w286) -> (element=w297:dbl)
          n87 = call-dynamic "Set External Attenuation.vi"("error in"=w289, "external attenuation (dB)"=w297, "device index (0)"=w286, "rtg api interface"=w300) -> ("error out"=w294:errorcluster, "rtg api interface out"=w299:refnum<class "NI-RTG Interface.lvclass">)  [unwired: 6 in]
          n88 = Index Array(array=w296, index=w286) -> (element=w295:dbl)
          n89 = call-dynamic "Set External Time Delay.vi"("error in"=w294, "delay (s)"=w295, "device index (0)"=w286, "rtg api interface"=w299) -> ("error out"=w293:errorcluster, "rtg api interface out"=w291:refnum<class "NI-RTG Interface.lvclass">)  [unwired: 6 in]
          n90 = Index Array(array=w288, index=w286) -> (element=w287:dbl)
          n91 = call-dynamic "Set Offset Frequency.vi"("error in"=w293, "offset frequency (Hz)"=w287, "device index (0)"=w286, "NI-RTG Interface in"=w291) -> ("error out"=w292:errorcluster, "NI-RTG Interface out"=w290:refnum<class "NI-RTG Interface.lvclass">)  [unwired: 6 in]
        }
        n92 = Bundle By Name(cluster=w281, "RTG Ref"=w271) -> (w280:T16)
        n93 = Merge Errors(w275) -> (w270:errorcluster)
        n94 = for {
          tunnel: w268 -> [w283]
          tunnel: cluster{"Enum":T3, "Var":variant}[] [{"Enum"=enum."RTG_GetCal", "Var"=variant}, {"Enum"=enum."RTG_SetPRIs", "Var"=variant}, {"Enum"=enum."RTG_CommAtten", "Var"=variant}] -> [w282] mode=indexing
          shift-right: [w284] -> w269
          shift-left: w270 -> [w285]
          n95 = Enqueue Element(queue=w283, element=w282, error in (no error)=w285) -> (error out=w284:errorcluster)  [unwired: 1 in, 2 out]
        }
      }
      frame "RTG_GetCal" {
        # "15. Return Calibrated RTG Minimums (Delay and Attenuation)"
        # "Get Calibration Data"
        n96 = Unbundle By Name(w311) -> ("VST_Names"=w310:string[], "RTG Ref"=w302:refnum<class "NI-RTG Interface.lvclass">)
        n97 = Array Size(array=w310) -> (size(s)=w303:i32)
        n98 = for {
          N: w303 -> [_]
          tunnel: w305 -> [w323]
          tunnel: [w320] -> w306 mode=indexing
          shift-right: [w318] -> w301
          shift-left: w302 -> [w321]
          tunnel: [w317] -> w309 mode=indexing
          tunnel: [w315] -> w307 mode=indexing
          tunnel: [w314] -> w308 mode=indexing
          i -> [w313]
          # "-------15-------"
          n99 = call-dynamic "Get Minimum Time Delay.vi"("error in"=w323, "device index (0)"=w313, "rtg api interface"=w321) -> ("error out"=w322:errorcluster, "delay (s)"=w317:dbl, "rtg api interface out"=w319:refnum<class "NI-RTG Interface.lvclass">)  [unwired: 5 in, 1 out]
          n100 = call-dynamic "Get Minimum Attenuations.vi"("error in"=w322, "device index (0)"=w313, "rtg api interface"=w319) -> ("error out"=w320:errorcluster, "attenuations (dB)"=w316:dbl[], "rtg api interface out"=w318:refnum<class "NI-RTG Interface.lvclass">)  [unwired: 5 in, 1 out]
          n101 = Array Max & Min(array=w316) -> (max value=w315:dbl, min value=w314:dbl)  [unwired: 2 out]
        }
        "Max Common Attenuations (dB)" <- w307
        "Min Common Attenuations (dB)" <- w308
        "Min Latencies (s)" <- w309
        n102 = Merge Errors(w306) -> (w304:errorcluster)
        n103 = Bundle By Name(cluster=w311, "RTG Ref"=w301) -> (w312:T16)
      }
      frame "RTG_SetPRIs" {
        n104 = Unbundle By Name(w331) -> ("RTG Ref"=w325:refnum<class "NI-RTG Interface.lvclass">)
        n105 = case shown="True" "Set PRIs" {
          tunnel: w325 -> [w333 w335]
          tunnel: [w333 w337] -> w324
          tunnel: w327 -> [w332 w334]
          tunnel: [w332 w336] -> w326
          tunnel: "PRI (s)" -> [_ w338]
          frame False {
          }
          frame True {
            n106 = for {
              tunnel: w338 -> [w344] mode=indexing
              shift-right: [w342] -> w337
              shift-left: w335 -> [w340]
              shift-right: [w341] -> w336
              shift-left: w334 -> [w339]
              i -> [w343]
              n107 = call-dynamic "Set PRI.vi"("error in"=w339, "pri (s)"=w344, "device index (0)"=w343, "NI-RTG Interface in"=w340) -> ("error out"=w341:errorcluster, "NI-RTG Interface out"=w342:refnum<class "NI-RTG Interface.lvclass">)  [unwired: 6 in]
            }
          }
        }
        n108 = Bundle By Name(cluster=w331, "RTG Ref"=w324) -> (w330:T16)
      }
      frame "RTG_CommAtten" {
        # "Begin regularly checking\nCoProcessor"
        # "17"
        n109 = Enqueue Element(queue=w345, element=cluster{"Enum":T2, "Data":variant} {"Enum"=enum."CoPr_Chk", "Data"=variant}, error in (no error)=w346) -> (error out=w347:errorcluster)  [unwired: 1 in, 2 out]
        n110 = Unbundle By Name(w361) -> ("RTG Ref"=w358:refnum<class "NI-RTG Interface.lvclass">, "Index"=w357:i32)
        n111 = call-dynamic "Set Common Attenuation.vi"("error in"=w347, "attenuation (dB)"="Common Attenuation (dB)", "device index (0)"=w357, "rtg api interface"=w358) -> ("error out"=w353:errorcluster, "rtg api interface out"=w356:refnum<class "NI-RTG Interface.lvclass">)  [unwired: 5 in, 1 out]
        n112 = Bundle By Name(cluster=w361, "RTG Ref"=w356) -> (w360:T16)
        n113 = To Variant(anything=Program_Status_Enum."RTG Inactive" ("Status")) -> (Variant=w350:variant)
        n114 = Bundle By Name(cluster=cluster{"Enum":T1, "Var":variant} {"Enum"=enum."Spvsr_UpdtFP", "Var"=variant}, "Var"=w350) -> (w354:cluster{"Enum":T1, "Var":variant})
        n115 = Enqueue Element(queue=w349, element=w354, error in (no error)=w353) -> (error out=w352:errorcluster)  [unwired: 1 in, 2 out]
      }
      frame "RTG_Start" {
        # "Starts the RTG running on the VST."
        n116 = Unbundle By Name(w369) -> ("RTG Ref"=w372:refnum<class "NI-RTG Interface.lvclass">)
        n117 = call-dynamic "Start.vi"("error in"=w373, "rtg api interface"=w372) -> ("error out"=w364:errorcluster, "rtg api interface out"=w371:refnum<class "NI-RTG Interface.lvclass">)  [unwired: 8 in]
        n118 = Bundle By Name(cluster=w369, "RTG Ref"=w371) -> (w370:T16)
        n119 = To Variant(anything=Program_Status_Enum."RTG active" ("Status")) -> (Variant=w365:variant)
        n120 = Bundle By Name(cluster=cluster{"Enum":T1, "Var":variant} {"Enum"=enum."Spvsr_UpdtFP", "Var"=variant}, "Var"=w365) -> (w367:cluster{"Enum":T1, "Var":variant})
        n121 = Enqueue Element(queue=w362, element=w367, error in (no error)=w364) -> (error out=w363:errorcluster)  [unwired: 1 in, 2 out]
      }
      frame "RTG_Stop" {
        # "The Stop is also used to end any current file transfer or target motion operation in progress."
        n122 = local write "Stop RTG"(FALSE ("Stop RTG")) -> ()
        n123 = Unbundle By Name(w385) -> ("RTG Ref"=w384:refnum<class "NI-RTG Interface.lvclass">)
        n124 = call-dynamic "Stop.vi"("error in"=w382, "rtg api interface"=w384) -> ("error out"=w376:errorcluster, "rtg api interface out"=w383:refnum<class "NI-RTG Interface.lvclass">)  [unwired: 8 in]
        n125 = Bundle By Name(cluster=w385, "RTG Ref"=w383) -> (w386:T16)
        n126 = To Variant(anything=Program_Status_Enum."RTG Inactive" ("Status")) -> (Variant=w377:variant)
        n127 = Bundle By Name(cluster=cluster{"Enum":T1, "Var":variant} {"Enum"=enum."Spvsr_UpdtFP", "Var"=variant}, "Var"=w377) -> (w379:cluster{"Enum":T1, "Var":variant})
        n128 = Enqueue Element(queue=w374, element=w379, error in (no error)=w376) -> (error out=w375:errorcluster)  [unwired: 1 in, 2 out]
      }
      frame "RTG_TargetSetup" {
        n129 = Bundle By Name(cluster=w390, "Index"="Device Index", "AutoSend"="Auto Send Software Trigger", "Prepend"="Prepend Software Trigger") -> (w391:T16)
      }
      frame "RTG_Send Target Cfg" {
        # "21"
        n130 = Unbundle By Name(w396) -> ("RTG Ref"=w397:refnum<class "NI-RTG Interface.lvclass">, "Index"=w393:i32)
        n131 = call-dynamic "Send Target Configuration.vi"("error in"=w399, "target config"="Target Configuration", "device index (0)"=w393, "rtg api interface"=w397) -> ("error out"=w398:errorcluster, "rtg api interface out"=w394:refnum<class "NI-RTG Interface.lvclass">)  [unwired: 5 in, 1 out]
        n132 = Bundle By Name(cluster=w396, "RTG Ref"=w394) -> (w395:T16)
      }
      frame "RTG_Send Files" {
        # "----------------------------------20----------------------------------"
        # "21"
        n133 = Unbundle By Name(w414) -> ("AutoSend"=w402:bool, "Prepend"=w401:bool, "RTG Ref"=w403:refnum<class "NI-RTG Interface.lvclass">, "Index"=w404:i32)
        n134 = case shown="True" w401 {
          tunnel: w403 -> [w423 w428]
          tunnel: w407 -> [w422 w425]
          tunnel: w404 -> [_ w427]
          tunnel: [w423 w426] -> w408
          tunnel: [w422 w424] -> w412
          frame False {
          }
          frame True {
            # "requires software trigger"
            n135 = call-dynamic "Send Target Configuration.vi"("error in"=w425, "target config"=T6 {"synchronization"={"synch mode"=enum."Software Trigger", "time offset (s)"=0.0}, "rtg targets"=[{"time offset (s)"=0.0, "attenuaton (dB)"=0.0, "doppler"=0.0, "target enable"=FALSE, "relative velocity enable"=FALSE}, {"time offset (s)"=0.0, "attenuaton (dB)"=0.0, "doppler"=0.0, "target enable"=FALSE, "relative velocity enable"=FALSE}, {"time offset (s)"=0.0, "attenuaton (dB)"=0.0, "doppler"=0.0, "target enable"=FALSE, "relative velocity enable"=FALSE}, {"time offset (s)"=0.0, "attenuaton (dB)"=0.0, "doppler"=0.0, "target enable"=FALSE, "relative velocity enable"=FALSE}]}, "device index (0)"=w427, "rtg api interface"=w428) -> ("error out"=w424:errorcluster, "rtg api interface out"=w426:refnum<class "NI-RTG Interface.lvclass">)  [unwired: 5 in, 1 out]
          }
        }
        n136 = call-dynamic "Send Target Configuration List - Files.vi"("error in"=w412, "target configuration file path"="Target Configuration Files", "device index (0)"=w404, "rtg api interface"=w408) -> ("error out"=w411:errorcluster, "rtg api interface out"=w410:refnum<class "NI-RTG Interface.lvclass">)  [unwired: 6 in]
        n137 = case shown="True" w402 {
          tunnel: w410 -> [w416 w421]
          tunnel: [w416 w420] -> w405
          tunnel: w411 -> [w415 w419]
          tunnel: [w415 w418] -> w406
          tunnel: w404 -> [_ w417]
          frame False {
          }
          frame True {
            n138 = call-dynamic "Send Software Trigger.vi"("error in"=w419, "device index (0)"=w417, "NI-RTG Interface in"=w421) -> ("error out"=w418:errorcluster, "NI-RTG Interface out"=w420:refnum<class "NI-RTG Interface.lvclass">)  [unwired: 7 in]
          }
        }
        n139 = Bundle By Name(cluster=w414, "RTG Ref"=w405) -> (w413:T16)
      }
      frame "RTG_Send Motion" {
        # "----------------------------22----------------------------"
        n140 = Unbundle By Name(w443) -> ("AutoSend"=w430:bool, "Prepend"=w431:bool, "RTG Ref"=w433:refnum<class "NI-RTG Interface.lvclass">, "Index"=w432:i32)
        n141 = case shown="True" w431 {
          tunnel: w433 -> [w452 w457]
          tunnel: w436 -> [w451 w454]
          tunnel: w432 -> [_ w456]
          tunnel: [w452 w455] -> w437
          tunnel: [w451 w453] -> w441
          frame False {
          }
          frame True {
            # "requires software trigger"
            n142 = call-dynamic "Send Target Configuration.vi"("error in"=w454, "target config"=T6 {"synchronization"={"synch mode"=enum."Software Trigger", "time offset (s)"=0.0}, "rtg targets"=[{"time offset (s)"=0.0, "attenuaton (dB)"=0.0, "doppler"=0.0, "target enable"=FALSE, "relative velocity enable"=FALSE}, {"time offset (s)"=0.0, "attenuaton (dB)"=0.0, "doppler"=0.0, "target enable"=FALSE, "relative velocity enable"=FALSE}, {"time offset (s)"=0.0, "attenuaton (dB)"=0.0, "doppler"=0.0, "target enable"=FALSE, "relative velocity enable"=FALSE}, {"time offset (s)"=0.0, "attenuaton (dB)"=0.0, "doppler"=0.0, "target enable"=FALSE, "relative velocity enable"=FALSE}]}, "device index (0)"=w456, "rtg api interface"=w457) -> ("error out"=w453:errorcluster, "rtg api interface out"=w455:refnum<class "NI-RTG Interface.lvclass">)  [unwired: 5 in, 1 out]
          }
        }
        n143 = call-dynamic "Send Target Configuration List - Target Motion.vi"("error in"=w441, "target motion parameters"="Target Motion Parameters", "device index (0)"=w432, "rtg api interface"=w437) -> ("error out"=w439:errorcluster, "rtg api interface out"=w438:refnum<class "NI-RTG Interface.lvclass">)  [unwired: 6 in]
        n144 = case shown="True" w430 {
          tunnel: w438 -> [w445 w450]
          tunnel: [w445 w449] -> w434
          tunnel: w439 -> [w444 w448]
          tunnel: [w444 w447] -> w435
          tunnel: w432 -> [_ w446]
          frame False {
          }
          frame True {
            n145 = call-dynamic "Send Software Trigger.vi"("error in"=w448, "device index (0)"=w446, "NI-RTG Interface in"=w450) -> ("error out"=w447:errorcluster, "NI-RTG Interface out"=w449:refnum<class "NI-RTG Interface.lvclass">)  [unwired: 7 in]
          }
        }
        n146 = Bundle By Name(cluster=w443, "RTG Ref"=w434) -> (w442:T16)
      }
      frame "RTG_Send SW Trigg" {
        n147 = Unbundle By Name(w465) -> ("RTG Ref"=w460:refnum<class "NI-RTG Interface.lvclass">, "Index"=w461:i32)
        n148 = call-dynamic "Send Software Trigger.vi"("error in"=w463, "device index (0)"=w461, "NI-RTG Interface in"=w460) -> ("error out"=w462:errorcluster, "NI-RTG Interface out"=w459:refnum<class "NI-RTG Interface.lvclass">)  [unwired: 7 in]
        n149 = Bundle By Name(cluster=w465, "RTG Ref"=w459) -> (w464:T16)
      }
      frame "RTG_Chk" {
        n150 = Wait Until Next ms Multiple(millisecond multiple=u32 100) -> ()  [unwired: 1 out]
        n151 = Enqueue Element(queue=w474, element=cluster{"Enum":T3, "Var":variant} {"Enum"=enum."RTG_Chk", "Var"=variant}, error in (no error)=w475) -> (error out=w476:errorcluster)  [unwired: 1 in, 2 out]
        n152 = Unbundle By Name(w480) -> ("RTG Ref"=w477:refnum<class "NI-RTG Interface.lvclass">)
        n153 = call-dynamic "Get Coprocessor Link Status.vi"("error in"=w476, "rtg api interface"=w477) -> ("error out"=w470:errorcluster, "rtg link status"=→"rtg link status":T12[], "rtg api interface out"=w468:refnum<class "NI-RTG Interface.lvclass">)  [unwired: 7 in]
        n154 = call-dynamic "Get RTG Status.vi"("error in"=w470, "rtg api interface"=w468) -> ("error out"=w469:errorcluster, "rtg status"=→"RTG Status":string, "state"=w466:T13, "rtg api interface out"=w467:refnum<class "NI-RTG Interface.lvclass">)  [unwired: 6 in]
        "RTG State" <- w466
        n155 = Bundle By Name(cluster=w480, "RTG Ref"=w467, "state"=w466) -> (w479:T16)
      }
      frame "RTG_Exit" {
        # "RTG Exit is called from Coprocesor Exit\nto prevent a race condition"
        n156 = Unbundle By Name(w482) -> ("RTG Ref"=w483:refnum<class "NI-RTG Interface.lvclass">)
        n157 = call-dynamic "Close.vi"("error in"=w485, "rtg api interface"=w483) -> ("error out"=w486:errorcluster, "rtg api interface out"=w487:refnum<class "NI-RTG Interface.lvclass">)  [unwired: 8 in]
        n158 = call-dynamic "Destroy.vi"("error in"=w486, "NI-RTG Interface in"=w487) -> ("error out"=w484:errorcluster)  [unwired: 9 in]
      }
    }
    n159 = call "Log_Errors_20190313.vi"("LoopName"="RTG", "error in"=w150) -> ("error out"=w149:errorcluster)  [unwired: 9 in]
    "RTG" <- w146
  }
  n160 = while {
    tunnel: w20 -> [w490]
    tunnel: w1 -> [w488]
    stop <- w489 stop-if-true
    # "Event Loop"
    n161 = event shown="[2] \"Commit HW\": Value Change" {
      selector: _ -> [_ _ _ _ _ _ _ _ _ _]
      dyn-events: _ -> [_ _ _ _ _ _ _ _ _ _]
      timeout: 200 -> [_ _ _ _ _ _ _ _ _ _]
      tunnel: w490 -> [_ _ w497 _ _ _ _ _ _ w526]
      tunnel: [_ _ _ _ _ _ _ _ _ TRUE] -> w489
      tunnel: w488 -> [_ w494 _ w502 w506 w510 w514 w518 w522 _]
      event Timeout {
        n162 = event-data() -> ()  [unwired: 1 in, 3 out]
        n163 = Get Date/Time String() -> (time string=→"System Time":string)  [unwired: 3 in, 1 out]
      }
      event "Start RTG": Value Change {
        n164 = event-data() -> ()  [unwired: 1 in, 6 out]
        n165 = Enqueue Element(queue=w494, element=cluster{"Enum":T3, "Var":variant} {"Enum"=enum."RTG_Start", "Var"=variant}) -> (error out=w495:errorcluster)  [unwired: 2 in, 2 out]
        n166 = call "Log_Errors_20190313.vi"("LoopName"="EventStart", "error in"=w495) -> ()  [unwired: 9 in, 1 out]
      }
      event "Commit HW": Value Change {
        n167 = event-data() -> ()  [unwired: 1 in, 6 out]
        n168 = Enqueue Element(queue=w497, element=cluster{"Enum":T1, "Var":variant} {"Enum"=enum."Spvsr_InitRTG", "Var"=variant}) -> (error out=w499:errorcluster)  [unwired: 2 in, 2 out]
        n169 = call "Log_Errors_20190313.vi"("LoopName"="EventStart", "error in"=w499) -> ()  [unwired: 9 in, 1 out]
      }
      event "Send SW Trigg": Value Change {
        n170 = event-data() -> ()  [unwired: 1 in, 6 out]
        n171 = Enqueue Element(queue=w502, element=cluster{"Enum":T3, "Var":variant} {"Enum"=enum."RTG_Send SW Trigg", "Var"=variant}) -> (error out=w503:errorcluster)  [unwired: 2 in, 2 out]
        n172 = call "Log_Errors_20190313.vi"("LoopName"="SW_Trigg", "error in"=w503) -> ()  [unwired: 9 in, 1 out]
      }
      event "Stop RTG": Value Change {
        n173 = event-data() -> ()  [unwired: 1 in, 6 out]
        n174 = Enqueue Element(queue=w506, element=cluster{"Enum":T3, "Var":variant} {"Enum"=enum."RTG_Stop", "Var"=variant}) -> (error out=w507:errorcluster)  [unwired: 2 in, 2 out]
        n175 = call "Log_Errors_20190313.vi"("LoopName"="EventStop", "error in"=w507) -> ()  [unwired: 9 in, 1 out]
      }
      event "Device Index", "Prepend Software Trigger", "Auto Send Software Trigger": Value Change {
        n176 = event-data() -> ()  [unwired: 1 in, 6 out]
        n177 = Enqueue Element(queue=w510, element=cluster{"Enum":T3, "Var":variant} {"Enum"=enum."RTG_TargetSetup", "Var"=variant}) -> (error out=w511:errorcluster)  [unwired: 2 in, 2 out]
        n178 = call "Log_Errors_20190313.vi"("LoopName"="DevIndex", "error in"=w511) -> ()  [unwired: 9 in, 1 out]
      }
      event "Send TrgtCfg": Value Change {
        n179 = event-data() -> ()  [unwired: 1 in, 6 out]
        n180 = Enqueue Element(queue=w514, element=cluster{"Enum":T3, "Var":variant} {"Enum"=enum."RTG_Send Target Cfg", "Var"=variant}) -> (error out=w515:errorcluster)  [unwired: 2 in, 2 out]
        n181 = call "Log_Errors_20190313.vi"("LoopName"="SendTargetCfg", "error in"=w515) -> ()  [unwired: 9 in, 1 out]
      }
      event "Send Motion": Value Change {
        n182 = event-data() -> ()  [unwired: 1 in, 6 out]
        n183 = Enqueue Element(queue=w518, element=cluster{"Enum":T3, "Var":variant} {"Enum"=enum."RTG_Send Motion", "Var"=variant}) -> (error out=w519:errorcluster)  [unwired: 2 in, 2 out]
        n184 = call "Log_Errors_20190313.vi"("LoopName"="SendMotion", "error in"=w519) -> ()  [unwired: 9 in, 1 out]
      }
      event "Send Files": Value Change {
        n185 = event-data() -> ()  [unwired: 1 in, 6 out]
        n186 = Enqueue Element(queue=w522, element=cluster{"Enum":T3, "Var":variant} {"Enum"=enum."RTG_Send Files", "Var"=variant}) -> (error out=w523:errorcluster)  [unwired: 2 in, 2 out]
        n187 = call "Log_Errors_20190313.vi"("LoopName"="SendFiles", "error in"=w523) -> ()  [unwired: 9 in, 1 out]
      }
      event "Exit": Value Change {
        n188 = event-data() -> ()  [unwired: 1 in, 6 out]
        n189 = To Variant(anything=Program_Status_Enum."Closing" ("Status")) -> (Variant=w527:variant)
        n190 = Bundle By Name(cluster=cluster{"Enum":T1, "Var":variant} {"Enum"=enum."Spvsr_UpdtFP", "Var"=variant}, "Var"=w527) -> (w529:cluster{"Enum":T1, "Var":variant})
        n191 = Enqueue Element(queue=w526, element=w529) -> (queue out=w525:refnum<queue>)  [unwired: 2 in, 2 out]
        n192 = Enqueue Element(queue=w525, element=cluster{"Enum":T1, "Var":variant} {"Enum"=enum."Spvsr_Exit", "Var"=variant}) -> (error out=w532:errorcluster)  [unwired: 2 in, 2 out]
        n193 = call "Log_Errors_20190313.vi"("LoopName"="EventExit", "error in"=w532) -> ()  [unwired: 9 in, 1 out]
      }
    }
  }
  n194 = while {
    tunnel: w12 -> [w547]
    tunnel: [w549] -> w4
    tunnel: w2 -> [w546]
    tunnel: w1 -> [w543]
    tunnel: w20 -> [w536]
    shift-right: [w542] -> _
    shift-left: T15 {"CoPr Refs"=[]} -> [w541]
    i -> [w535]
    stop <- w537 stop-if-true
    # "CoProcessor Loop"
    n195 = Dequeue Element(queue=w546, error in (no error)=w547) -> (queue out=w538:refnum<queue>, element=w548:cluster{"Enum":T2, "Data":variant}, error out=w540:errorcluster)  [unwired: 1 in, 1 out]
    n196 = Unbundle(w548) -> ("Enum"=w545:T2, "Data"=w544:variant)
    "CoPr" <- w545
    n197 = case shown="\"CoPr_Chk\"" w545 {
      tunnel: w544 -> [w564 _ _]
      tunnel: w543 -> [w559 _ w621]
      tunnel: [w568 w584 w624] -> w542
      tunnel: w541 -> [w567 w584 w624]
      tunnel: w540 -> [w565 w593 w619]
      tunnel: [w560 w582 w626] -> w539
      tunnel: w538 -> [_ w592 _]
      tunnel: [_ _ TRUE] -> w537
      tunnel: w536 -> [_ w581 _]
      frame "CoPr_Init" {
        # "3. Create and Intialize Coprocessor Object if valid Coprocessor Hardware"
        # "3"
        n198 = Variant To Data(error in=w565, type="" ("option string"), Variant=w564) -> (data=w562:string, error out=w566:errorcluster)
        n199 = call <vilib>:"Create Coprocessor.vi"("error in"=w566, "option string"=w562, "coprocessor resources"="Coprocessor Names") -> ("error out"=w561:errorcluster, "rtg coprocessor links"=w556:refnum<class "RTG Coprocessor Link Interface.lvclass">[])  [unwired: 7 in]
        n200 = Bundle By Name(cluster=w567, "CoPr Refs"=w556) -> (w568:T15)
        n201 = To Variant(anything=w556) -> (Variant=w555:variant)
        n202 = Bundle By Name(cluster=cluster{"Enum":T3, "Var":variant} {"Enum"=enum."RTG_RefLvl", "Var"=variant}, "Var"=w555) -> (w557:cluster{"Enum":T3, "Var":variant})
        n203 = Build Array(w557, cluster{"Enum":T3, "Var":variant} {"Enum"=enum."RTG_mmWav", "Var"=variant}, cluster{"Enum":T3, "Var":variant} {"Enum"=enum."RTG_Cal", "Var"=variant}, cluster{"Enum":T3, "Var":variant} {"Enum"=enum."RTG_CalDone?", "Var"=variant}) -> (w554:cluster{"Enum":T3, "Var":variant}[])
        n204 = for {
          tunnel: w559 -> [w571]
          tunnel: w554 -> [w570] mode=indexing
          shift-right: [w572] -> w560
          shift-left: w561 -> [w573]
          n205 = Enqueue Element(queue=w571, element=w570, error in (no error)=w573) -> (error out=w572:errorcluster)  [unwired: 1 in, 2 out]
        }
      }
      frame "CoPr_Chk" {
        # "Send count\nwhen it \nchanges"
        n206 = Unbundle By Name(w584) -> ("CoPr Refs"=w585:refnum<class "RTG Coprocessor Link Interface.lvclass">[])
        n207 = Wait Until Next ms Multiple(millisecond multiple=u32 100) -> ()  [unwired: 1 out]
        n208 = Enqueue Element(queue=w592, element=cluster{"Enum":T2, "Data":variant} {"Enum"=enum."CoPr_Chk", "Data"=variant}, error in (no error)=w593) -> (error out=w586:errorcluster)  [unwired: 1 in, 2 out]
        n209 = for {
          tunnel: w585 -> [w606] mode=indexing
          tunnel: [w610] -> w587 mode=indexing
          shift-right: [w603] -> w583
          shift-left: w586 -> [w611]
          tunnel: [w605] -> w589 mode=indexing
          tunnel: [w599] -> w588 mode=indexing
          n210 = call-dynamic "Get Coprocessor Refnum.vi"("rtg coprocessor link interface"=w606) -> ("error out"=w609:errorcluster, "coprocessor refnum"=w607:refnum<k20>)  [unwired: 8 in, 1 out]
          n211 = call-dynamic "Coprocessor Link Status.vi"("error in"=w611, "rtg coprocessor link interface"=w606) -> ("error out"=w601:errorcluster, "coprocessor status out"=w610:T14, "rtg coprocessor link interface out"=w602:refnum<class "RTG Coprocessor Link Interface.lvclass">)  [unwired: 7 in]
          n212 = Not A Number/Path/Refnum?(number/path/refnum=w607) -> (NaN/Path/Refnum?=w608:bool)
          n213 = case shown="False" w608 {
            tunnel: w607 -> [w615 _]
            tunnel: w609 -> [w614 w618]
            tunnel: [w613 w618] -> w604
            tunnel: [w612 _] -> w605
            frame False {
              # "Read RTG coprocessor \nrecieved trigger count"
              n214 = Dynamic FPGA Interface Cast(Session In=refnum<k20> refnum ("Type"), Type=w615) -> (Session Out=w617:refnum<k20>)
              n215 = xnode "Read/Write Control"("FPGA VI Reference In"=w617, "error in"=w614) -> ("error out"=w613:errorcluster, "read trigger rising edge count"=w612:u16)  [unwired: 1 out]
            }
            frame True {
            }
          }
          n216 = call-dynamic "Get Device Index.vi"("error in"=w601, "rtg coprocessor link interface"=w602) -> ("error out"=w600:errorcluster, "device index"=w599:i32)  [unwired: 7 in, 1 out]
          n217 = Merge Errors(w600, w604) -> (w603:errorcluster)
        }
        "coproc link" <- w587
        n218 = Build Array(w588, w589) -> (w575:i32[][])
        n219 = feedback-in #1(w575) -> ()
        n220 = feedback #1(i32[][] []) -> (w576:i32[][])
        n221 = To Variant(anything=w575) -> (Variant=w578:variant)
        n222 = Not Equal?(x=w575, y=w576) -> (x != y?=w574:bool)
        n223 = Bundle By Name(cluster=cluster{"Enum":T1, "Var":variant} {"Enum"=enum."Spvsr_StateCount", "Var"=variant}, "Var"=w578) -> (w579:cluster{"Enum":T1, "Var":variant})
        n224 = case shown="True" w574 {
          tunnel: w583 -> [w594 w598]
          tunnel: [w594 w597] -> w582
          tunnel: w581 -> [_ w596]
          tunnel: w579 -> [_ w595]
          frame False {
          }
          frame True {
            n225 = Enqueue Element(queue=w596, element=w595, error in (no error)=w598) -> (error out=w597:errorcluster)  [unwired: 1 in, 2 out]
          }
        }
      }
      frame "CoPr_Exit" {
        n226 = Enqueue Element(queue=w621, element=cluster{"Enum":T3, "Var":variant} {"Enum"=enum."RTG_Exit", "Var"=variant}, error in (no error)=w619) -> (error out=w620:errorcluster)  [unwired: 1 in, 2 out]
        n227 = Unbundle By Name(w624) -> ("CoPr Refs"=w625:refnum<class "RTG Coprocessor Link Interface.lvclass">[])
        n228 = for {
          tunnel: w625 -> [w629] mode=indexing
          shift-right: [w627] -> w626
          shift-left: w620 -> [w628]
          # "29"
          n229 = call-dynamic "Close.vi"("error in"=w628, "rtg coprocessor link interface"=w629) -> ("error out"=w627:errorcluster)  [unwired: 9 in]
        }
      }
    }
    n230 = call "Log_Errors_20190313.vi"("LoopName"="CoPr", "error in"=w539) -> ("error out"=w549:errorcluster)  [unwired: 9 in]
    "CoPr" <- w535
  }
  n231 = flat-sequence {
    tunnel: w20 -> [w641]
    tunnel: w6 -> [w640]
    tunnel: w5 -> [w639]
    tunnel: w4 -> [w638]
    tunnel: w2 -> [w636]
    tunnel: w1 -> [w635]
    frame #0 {
      w634 = FALSE ("Stop RTG")
      n232 = Release Queue(queue=w641) -> (error out=w631:errorcluster)  [unwired: 2 in, 2 out]
      n233 = Release Queue(queue=w635) -> (error out=w632:errorcluster)  [unwired: 2 in, 2 out]
      n234 = Release Queue(queue=w636) -> (error out=w633:errorcluster)  [unwired: 2 in, 2 out]
      n235 = Merge Errors(w631, w632, w633, w640, w639, w638) -> (w637:errorcluster)
      n236 = local write "error out"(w637) -> ()
      n237 = local write "App Status"(Program_Status_Enum."Closed" ("App Status")) -> ()
      n238 = local write "Stop RTG"(w634) -> ()
      n239 = local write "Exit"(w634) -> ()
    }
  }
